vi "log_in_file.vi"(0 "file path":path, 1 "save?":bool, 2 "mm:ss":string, 3 "temperature":dbl, 4 "capacity":dbl, 5 "current":dbl, 6 "voltage":dbl) -> ()   [LabVIEW 2016]
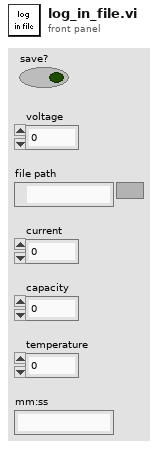
[diagram p1: front panel]
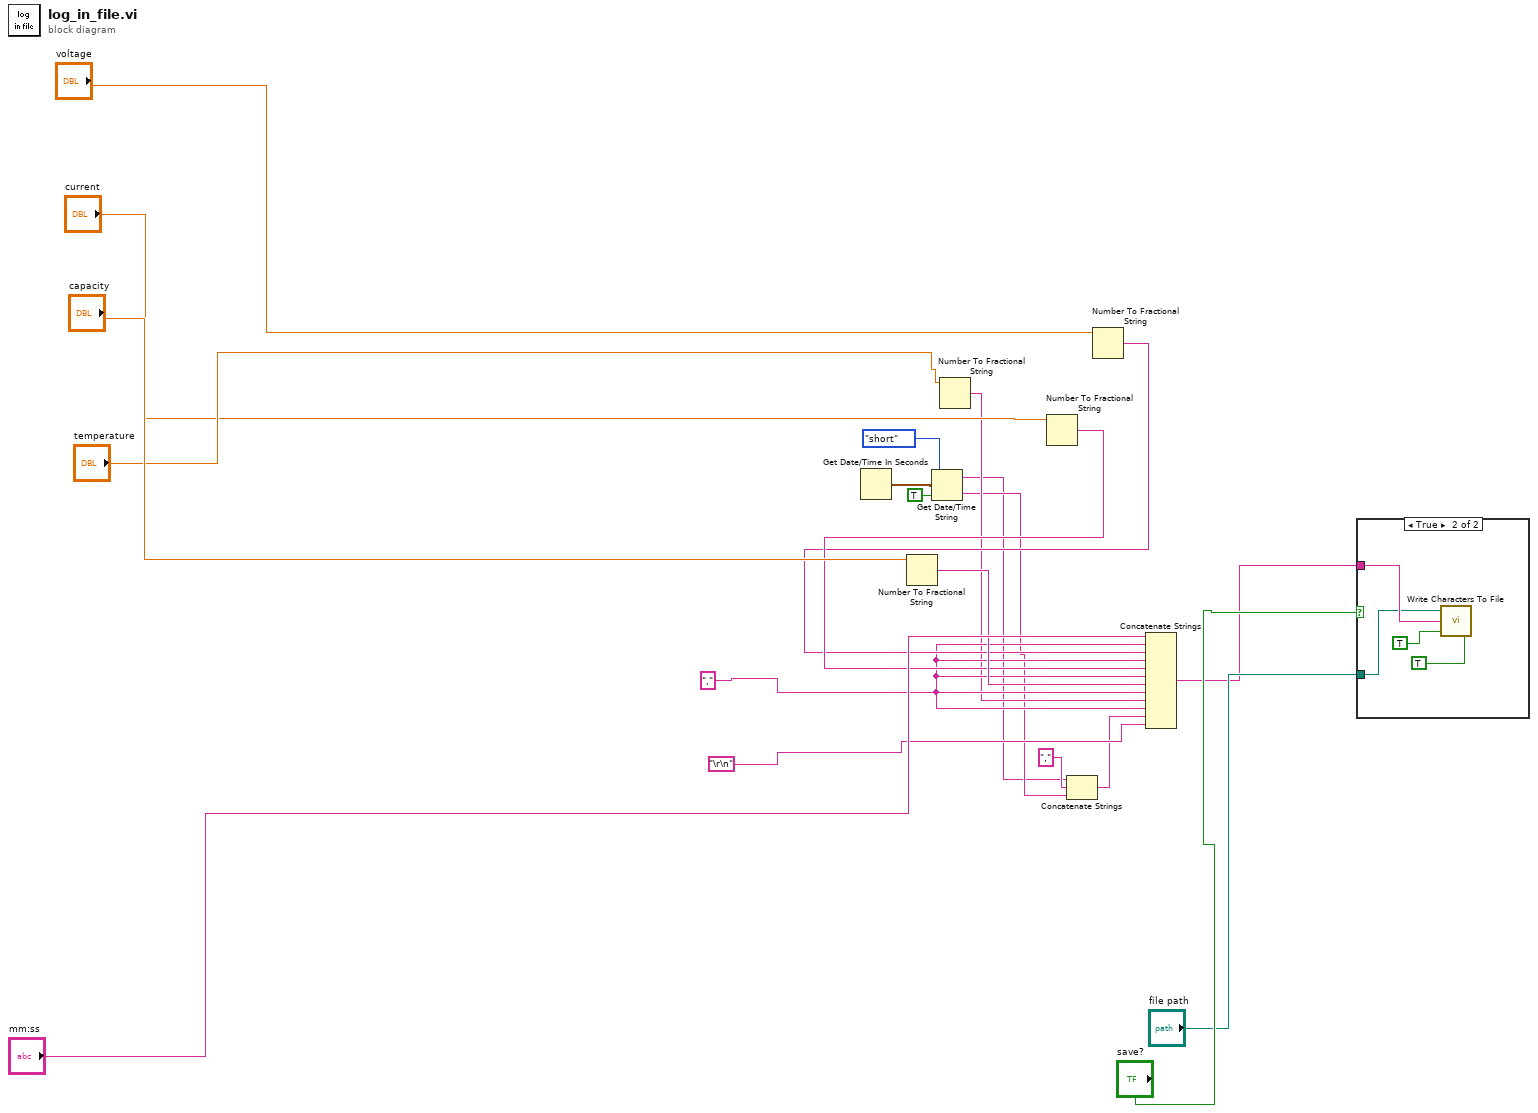
[diagram p0: block diagram]
diagram:
  w13 = "," ("string")
  n1 = Get Date/Time In Seconds() -> (seconds since 1Jan1904=w2:timestamp)
  n2 = Number To Fractional String(number="capacity") -> (F-format string=w16:string)  [unwired: 3 in]
  n3 = Get Date/Time String(date format (0)=enum16{"short", "long", "abbreviated"}."short", seconds (now)=w2, want seconds? (F)=TRUE) -> (date string=w5:string, time string=w6:string)
  n4 = Number To Fractional String(number="temperature") -> (F-format string=w9:string)  [unwired: 3 in]
  n5 = Number To Fractional String(number="current") -> (F-format string=w15:string)  [unwired: 3 in]
  n6 = Concatenate Strings(w5, "," ("string"), w6) -> (w10:string)
  n7 = Number To Fractional String(number="voltage") -> (F-format string=w14:string)  [unwired: 3 in]
  n8 = Concatenate Strings("mm:ss", w13, w14, w13, w15, w13, w16, w13, w9, w13, w10, "\r\n") -> (w1:string)
  n9 = case shown="True" "save?" {
    tunnel: w1 -> [_ w25]
    tunnel: "file path" -> [_ w22]
    frame False {
    }
    frame True {
      n10 = call <vilib>:"Write Characters To File.vi"("convert eol? (no:F)"=TRUE, "append to file? (new file:F)"=TRUE, "character string"=w25, "file path (dialog if empty)"=w22) -> ()  [unwired: 1 in, 1 out]
    }
  }
